vi "simpleCounterGlobals.vi"() -> ()   [LabVIEW 2014]
panel:
  out "simpleCounterWriteOverflow":bool
  in  "stop":bool
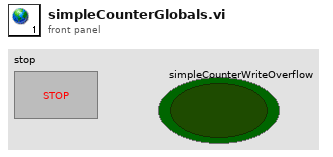
[diagram p1: front panel]
diagram:
